vi "goto location.vi"(0 "Image Data":T1) -> (1 "left speed":dbl, 2 "right speed":dbl)   [LabVIEW 2013]
uses:
  typedefs/vision data.ctl
  <vilib>/addons/control/pid/pid.llb/PID (DBL).vi
  <vilib>/addons/control/pid/NI_PID_pid.lvlib
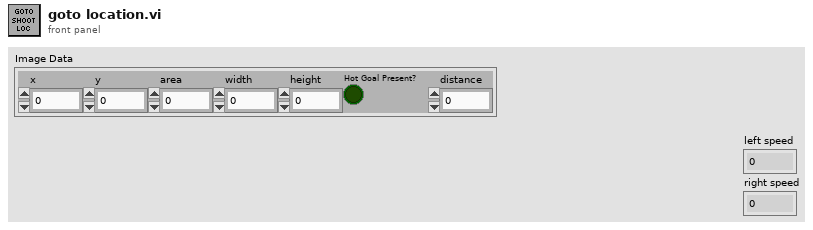
[diagram p1: front panel]
types:
  T1 = typedef "vision data.ctl" = cluster{"x":dbl, "y":dbl, "area":dbl, "width":dbl, "height":dbl, "Hot Goal Present?":bool, "distance":dbl}
  T2 = cluster{"proportional gain (Kc)":dbl, "integral time (Ti, min)":dbl, "derivative time (Td, min)":dbl}
  T3 = typedef "WPI_EncoderDevRef.ctl" = cluster{"DevStatus":errorcluster, "EncoderIndex":T4, "CounterIndex":T5, "DistancePerCount":dbl, "Decoding Type":T6}
  T4 = typedef "FPGA_EncoderIdx.ctl" = enum8{"Enc 0", "Enc 1", "Enc 2", "Enc 3", "Invalid"}
  T5 = typedef "FPGA_CounterCtrSystemIndex.ctl" = enum8{"Ctr 0", "Ctr 1", "Ctr 2", "Ctr 3", "Ctr 4", "Ctr 5", "Ctr 6", "Ctr 7", "Invalid"}
  T6 = typedef "WPI_EncoderType.ctl" = enum16{"1x", "2x", "4x"}
  T7 = cluster{"x":bool, "y":bool, "area":bool, "width":bool, "height":bool, "Hot Goal Present?":bool, "distance":bool}
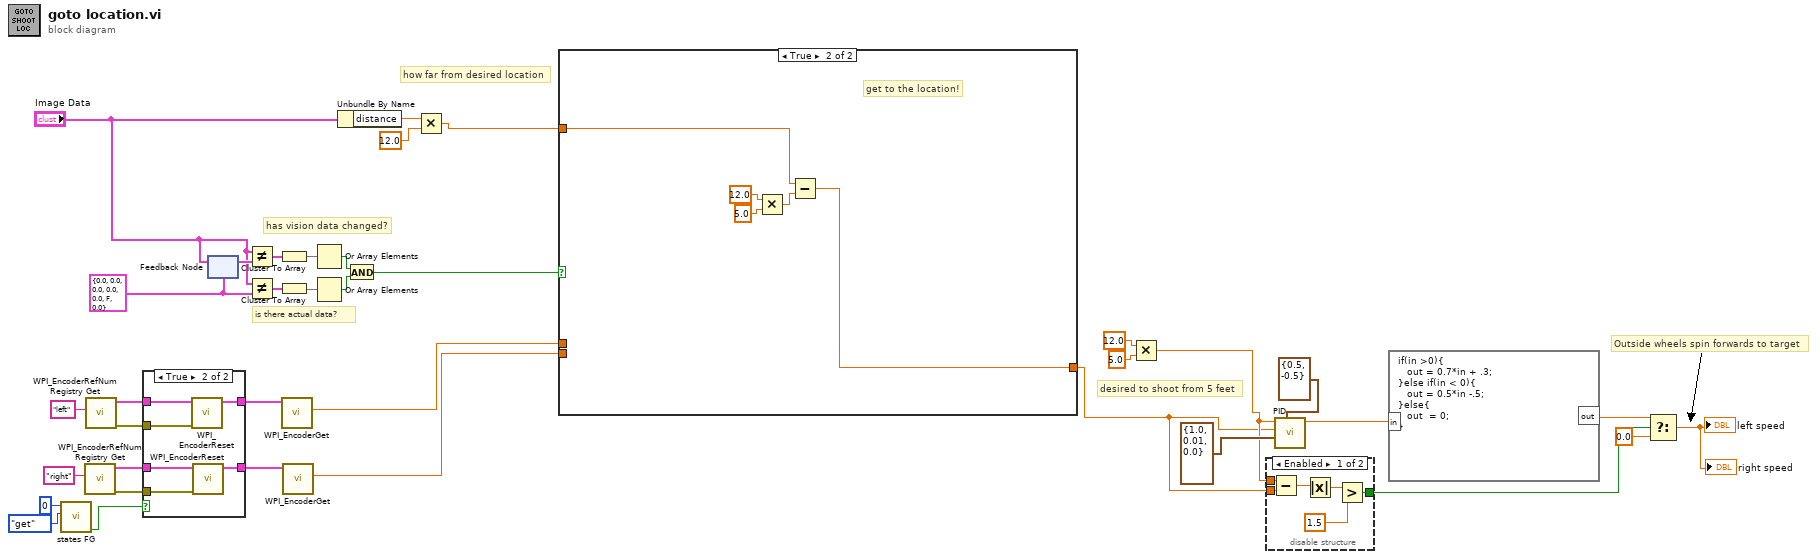
[diagram p0: block diagram]
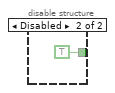
[diagram p2: hidden frame]
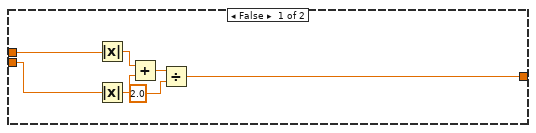
[diagram p3: hidden frame]
diagram:
  w29 = T1 {"x"=0.0, "y"=0.0, "area"=0.0, "width"=0.0, "height"=0.0, "Hot Goal Present?"=FALSE, "distance"=0.0} ("Image Data")
  # "Outside wheels spin forwards to target"
  # "how far from desired location"
  # "desired to shoot from 5 feet"
  # "is there actual data?"
  # "has vision data changed?"
  n1 = call "states FG.vi"("menu (get)"=enum16{"set", "get"}."get", "Loop ID"=0) -> ("first call?"=w20:bool)  [unwired: 6 in, 3 out]
  n2 = call <vilib>:"WPI_EncoderRefNum Registry Get.vi"("refnum name"="right") -> ("error out"=w23:errorcluster, "EncoderDevRef"=w24:T3)  [unwired: 9 in]
  n3 = call <vilib>:"WPI_EncoderRefNum Registry Get.vi"("refnum name"="left") -> ("error out"=w25:errorcluster, "EncoderDevRef"=w26:T3)  [unwired: 9 in]
  n4 = case shown="True" w20 {
    tunnel: w26 -> [w39 w45]
    tunnel: w25 -> [_ w44]
    tunnel: w24 -> [w38 w43]
    tunnel: w23 -> [_ w42]
    tunnel: [w39 w41] -> w22
    tunnel: [w38 w40] -> w21
    frame False {
    }
    frame True {
      n5 = call <vilib>:"WPI_EncoderReset.vi"("error in (no error)"=w44, "EncoderDevRef"=w45) -> ("EncoderDevRef"=w41:T3)  [unwired: 8 in, 1 out]
      n6 = call <vilib>:"WPI_EncoderReset.vi"("error in (no error)"=w42, "EncoderDevRef"=w43) -> ("EncoderDevRef"=w40:T3)  [unwired: 8 in, 1 out]
    }
  }
  n7 = feedback #1(w29) -> (w34:T1)
  n8 = feedback-in #1("Image Data") -> ()
  n9 = Not Equal?(x="Image Data", y=w34) -> (x != y?=w37:T7)
  n10 = Not Equal?(x="Image Data", y=w29) -> (x != y?=w35:T7)
  n11 = Cluster To Array(cluster=w37) -> (array=w36:bool[])
  n12 = Cluster To Array(cluster=w35) -> (array=w32:bool[])
  n13 = call <vilib>:"WPI_EncoderGet.vi"("EncoderDevRef"=w22) -> ("Distance"=w14:dbl)  [unwired: 5 in, 5 out]
  n14 = call <vilib>:"WPI_EncoderGet.vi"("EncoderDevRef"=w21) -> ("Distance"=w13:dbl)  [unwired: 5 in, 5 out]
  n15 = Or Array Elements(Boolean array=w36) -> (logical OR=w33:bool)
  n16 = Or Array Elements(Boolean array=w32) -> (logical OR=w31:bool)
  n17 = Unbundle By Name("Image Data") -> ("distance"=w16:dbl)
  n18 = And(x=w33, y=w31) -> (x .and. y?=w17:bool)
  n19 = Multiply(x=w16, y=12.0) -> (x*y=w4:dbl)
  n20 = case shown="True" w17 {
    tunnel: w14 -> [w48 _]
    tunnel: w13 -> [w47 _]
    tunnel: w4 -> [_ w54]
    tunnel: [w46 w53] -> w1
    frame False {
      n21 = Absolute Value(x=w48) -> (abs(x)=w49:dbl)
      n22 = Absolute Value(x=w47) -> (abs(x)=w50:dbl)
      n23 = Add(x=w49, y=w50) -> (x+y=w51:dbl)
      n24 = Divide(x=w51, y=2.0) -> (x/y=w46:dbl)
    }
    frame True {
      # "get to the location!"
      n25 = Multiply(x=12.0 ("y"), y=5.0) -> (x*y=w55:dbl)
      n26 = Subtract(x=w54, y=w55) -> (x-y=w53:dbl)
    }
  }
  n27 = Multiply(x=12.0 ("y"), y=5.0) -> (x*y=w2:dbl)
  n28 = disable-structure shown="Enabled" {
    disable-tunnel: w1 -> [w62 _]
    disable-tunnel: [w59 TRUE] -> w5
    disable-tunnel: w2 -> [w58 _]
    frame Enabled {
      n29 = Subtract(x=w58, y=w62) -> (x-y=w63:dbl)
      n30 = Absolute Value(x=w63) -> (abs(x)=w61:dbl)
      n31 = Greater?(x=w61, y=1.5) -> (0:w59:bool)
    }
    frame Disabled {
    }
  }
  n32 = call-poly <vilib>:"PID.vi"("output range"=cluster{"output high":dbl, "output low":dbl} {"output high"=0.5, "output low"=-0.5}, "PID gains"=T2 {"proportional gain (Kc)"=1.0, "integral time (Ti, min)"=0.01, "derivative time (Td, min)"=0.0}, "process variable"=w1, "setpoint"=w2) -> ("output"=w9:dbl)  [unwired: 6 in, 1 out]
  n33 = formula code="if(in >0){\n   out = 0.7*in + .3;\n}else if(in < 0){\n   out = 0.5*in -.5;\n}else{\n   out  = 0;\n}"("in"=w9) -> ("out"=w10:dbl)
  n34 = Select(t=w10, s=w5, f=0.0) -> (s? t:f=→"left speed" →"right speed":dbl)
